vi "Edit Community Link Flags.vi"   [LabVIEW 2020]
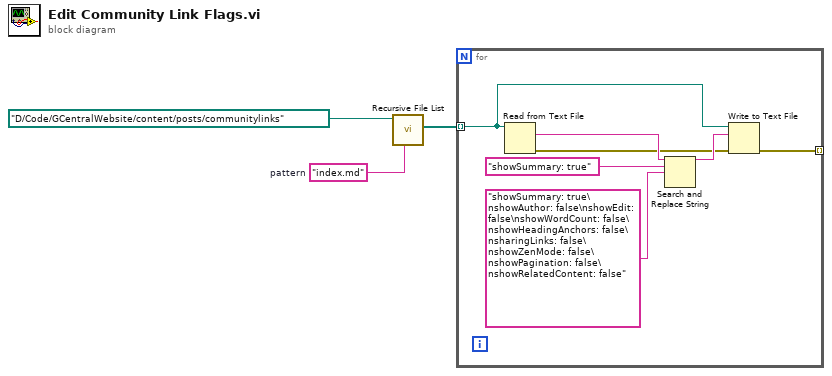
[diagram p0: block diagram]
diagram:
  w2 = "index.md"  # pattern
  n1 = call <vilib>:"Recursive File List.vi"("pattern"=w2, "Folder Path"=path "D:/Code/GCentralWebsite/content/posts/communitylinks") -> ("All Files in Dir"=w1:path[])  [unwired: 5 in, 4 out]
  n2 = for {
    tunnel: w1 -> [w4] mode=indexing
    tunnel: [w6] -> _ mode=indexing
    n3 = Read from Text File(file (use dialog)=w4) -> (text=w10:string, error out=w5:errorcluster)  [unwired: 3 in, 2 out]
    n4 = Search and Replace String(input string=w10, search string="showSummary: true", replace string="showSummary: true\nshowAuthor: false\nshowEdit: false\nshowWordCount: false\nshowHeadingAnchors: false\nsharingLinks: false\nshowZenMode: false\nshowPagination: false\nshowRelatedContent: false") -> (result string=w8:string)  [unwired: 5 in, 3 out]
    n5 = Write to Text File(file (use dialog)=w4, text=w8, error in=w5) -> (error out=w6:errorcluster)  [unwired: 1 in, 2 out]
  }
